vi "DirectionChange.vi"(8 "error in (no error)":errorcluster, 10 "New Direction":T1, 11 "Game Data in":T2) -> (0 "error out":errorcluster, 3 "Game Data out":T2)   [LabVIEW 2020]
uses:
  TypeDef/game-data.ctl
  TypeDef/tiles-key.ctl
  TypeDef/direction.ctl
  <vilib>/Utility/error.llb/Error Cluster From Error Code.vi
  <vilib>/ErrorRing/Error Ring.xnode
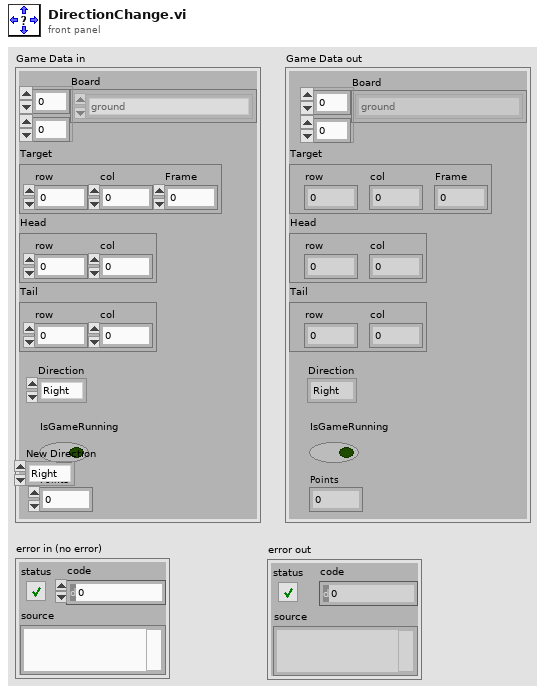
[diagram p1: front panel]
types:
  T1 = typedef "direction.ctl" = enum16{"Right", "Up", "Left", "Down"}
  T2 = typedef "game-data.ctl" = cluster{"Board":T3[][], "Target":cluster{"row":i32, "col":i32, "Frame":i8}, "Head":cluster{"row":i32, "col":i32}, "Tail":cluster{"row":i32, "col":i32}, "Direction":T1, "IsGameRunning":bool, "Points":i32}
  T3 = typedef "tiles-key.ctl" = enum16{"ground", "wall", "head (right)", "head (up)", "head (left)", "head (down)", "L-turn (right-up)", "L-turn (up-left)", "L-turn (left-down)", "L-turn (down-right)", "body (right)", "body (up)", "body (left)", "body (down)", "R-turn (right-down)", "R-turn (up-right)", "R-turn (left-up)", "R-turn (down-left)", "tail (right)", "tail (up)", "tail (left)", "tail (down)", "dead head (right)", "dead head (up)", "dead head (left)", "dead head (down)", "dead L-turn (right-up)", "dead L-turn (up-left)", "dead L-turn (left-down)", "dead L-turn (down-right)", "dead body (right)", "dead body (up)", "dead body (left)", "dead body (down)", "dead R-turn (right-down)", "dead R-turn (up-right)", "dead R-turn (left-up)", "dead R-turn (down-left)", "dead tail (right)", "dead tail (up)", "dead tail (left)", "dead tail (down)", "target red", "target blue", "target yellow", "target green"}
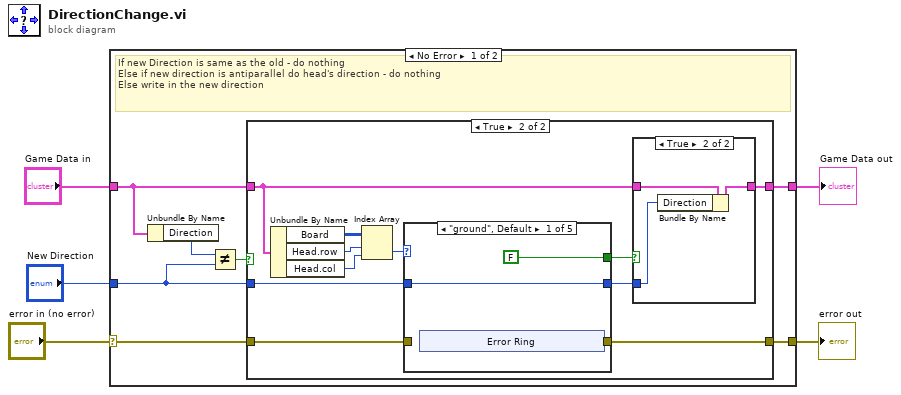
[diagram p0: block diagram]
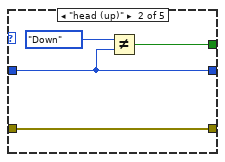
[diagram p4: hidden frame]
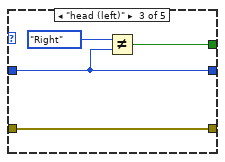
[diagram p5: hidden frame]
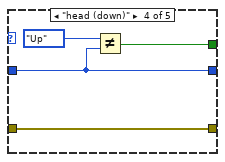
[diagram p6: hidden frame]
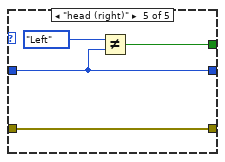
[diagram p7: hidden frame]
diagram:
  n1 = case shown="No Error" "error in (no error)" {
    selector: "error in (no error)" -> [w7 w55]
    tunnel: [w6 w55] -> w4
    tunnel: "Game Data in" -> [w12 w54]
    tunnel: "New Direction" -> [w9 _]
    tunnel: [w8 w54] -> w1
    frame No Error {
      # "If new Direction is same as the old - do nothing\nElse if new direction is antiparallel do head's direction - do nothing\nElse write in the new direction"
      n2 = Unbundle By Name(w12) -> ("Direction"=w10:T1)
      n3 = Not Equal?(x=w10, y=w9) -> (x != y?=w11:bool)
      n4 = case shown="True" w11 {
        tunnel: w12 -> [w14 w17]
        tunnel: w9 -> [_ w19]
        tunnel: [w14 w16] -> w8
        tunnel: w7 -> [w13 w22]
        tunnel: [w13 w21] -> w6
        frame False {
        }
        frame True {
          n5 = Unbundle By Name(w17) -> ("Board"=w25:T3[][], "Head.row"=w24:i32, "Head.col"=w20:i32)
          n6 = Index Array(array=w25, index (row)=w24, index (col)=w20) -> (element=w23:T3)
          n7 = case shown="\"ground\", Default" w23 {
            tunnel: w22 -> [_ w41 w45 w49 w53]
            tunnel: [w32 w41 w45 w49 w53] -> w21
            tunnel: w19 -> [w31 w39 w42 w46 w50]
            tunnel: [w31 w39 w42 w46 w50] -> w15
            tunnel: [FALSE w38 w44 w48 w52] -> w18
            frame "ground", Default {
              n8 = xnode "Error Ring"() -> ("error out"=w32:errorcluster)
            }
            frame "head (up)" {
              n9 = Not Equal?(x=direction."Down" ("Direction"), y=w39) -> (x != y?=w38:bool)
            }
            frame "head (left)" {
              n10 = Not Equal?(x=direction."Right" ("Direction"), y=w42) -> (x != y?=w44:bool)
            }
            frame "head (down)" {
              n11 = Not Equal?(x=direction."Up" ("Direction"), y=w46) -> (x != y?=w48:bool)
            }
            frame "head (right)" {
              n12 = Not Equal?(x=direction."Left" ("Direction"), y=w50) -> (x != y?=w52:bool)
            }
          }
          n13 = case shown="True" w18 {
            tunnel: w17 -> [w26 w29]
            tunnel: [w26 w28] -> w16
            tunnel: w15 -> [_ w27]
            frame False {
            }
            frame True {
              n14 = Bundle By Name(cluster=w29, "Direction"=w27) -> (w28:T2)
            }
          }
        }
      }
    }
    frame Error {
    }
  }
  "Game Data out" <- w1
  "error out" <- w4
